vi "Data to Single Line String_Do.vi"(8 "error in (no error)":errorcluster, 11 "System Exec Data in":refnum<class "System Exec Data.lvclass">) -> (0 "error out":errorcluster, 3 "String Data":string)   [LabVIEW 2020, in "ProjectBuilder.lvlib" / "System Exec Data.lvclass"]
doc: "Format private data into a string.\n\nThis implementation creates the following string:\n[Start Time] Action name ([alias ]): [Success or Failed (code)]"
uses:
  System Exec Data.lvclass
  Data/Report Data/Report Data.lvclass
  PPL/HDH.ClassLoader.lvlibp
  C:/Current projects/WS/LV32.2020..ProjectBuilder/Class/Data/Report Data/Report Data.lvclass
  C:/Current projects/WS/LV32.2020..ProjectBuilder/Class/Run System Exec/System Exec Data/System Exec Data.lvclass
  Project Action/Project Action.lvclass
  C:/Current projects/WS/LV32.2020..ProjectBuilder/Class/Project Action/Project Action.lvclass
  C:/Current projects/WS/LV32.2020..ProjectBuilder/Interface/Action Interface/Action Interface.lvclass
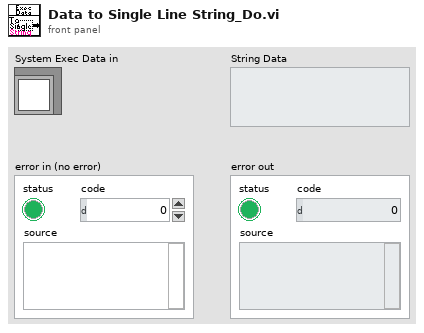
[diagram p1: front panel]
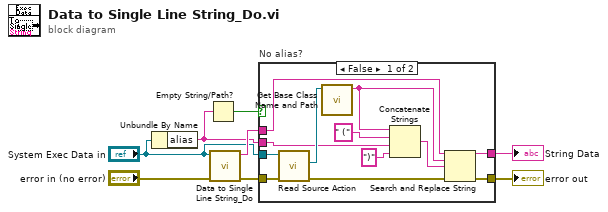
[diagram p0: block diagram]
diagram:
  n1 = Unbundle By Name("System Exec Data in") -> ("alias"=w3:string)
  n2 = Empty String/Path?(string/path=w3) -> (empty?=w7:bool)
  n3 = call-parent "Data to Single Line String_Do.vi"("error in (no error)"="error in (no error)", "Report Data in"="System Exec Data in") -> ("error out"=w1:errorcluster, "String Data"=w5:string)  [unwired: 8 in]
  n4 = case "No alias?" shown="False" w7 {
    tunnel: [w9 w22] -> w6
    tunnel: w5 -> [w18 w22]
    tunnel: "System Exec Data in" -> [w20 _]
    tunnel: w3 -> [w15 _]
    tunnel: [w10 w21] -> w2
    tunnel: w1 -> [w12 w21]
    frame False {
      n5 = call "Read Source Action.vi"("error in (no error)"=w12, "Report Data in"=w20) -> ("error out"=w11:errorcluster, "Source Action"=w19:refnum<class "Project Action.lvclass">)  [unwired: 7 in, 1 out]
      n6 = call "Get Base Class Name and Path.vi"("Class"=w19) -> ("Base Class Name"=w17:string)  [unwired: 8 in, 2 out]
      n7 = Concatenate Strings(w17, " (" ("string"), w15, ")" ("string")) -> (w13:string)
      n8 = Search and Replace String(input string=w18, search string=w17, replace string=w13, error in=w11) -> (result string=w9:string, error out=w10:errorcluster)  [unwired: 4 in, 2 out]
    }
    frame True {
    }
  }
  "error out" <- w2
  "String Data" <- w6
